vi "IBM4_Diff_Read(I1).vi"(8 "error in":errorcluster, 9 "Neg-Chan":i32=1, 10 "Pos-Chan":i32, 11 "COM resource in":refnum<visa-resource-name>="COM9") -> (0 "error out":errorcluster, 2 "output":i32, 3 "COM resource out":refnum<visa-resource-name>)   [LabVIEW 2021, in "IBM4.lvlib"]
doc: "This VI interfaces with the IBM4 to perform a differential read operation.\n\nThe input channels must be between 0 and 4, while the output will in binary format (thus, integer).\nOnly a single read operation is made with this VI. \n\nAlternate read operations exist covering binary or floating point, single reading, multiple readings, and an average of multiple readings (floating point only)."
uses:
  IBM4.lvlib
  <vilib>/Instr/_visa.llb/VISA Configure Serial Port (Instr).vi
panel:
  out "error out 2":errorcluster
  out "read buffer":string
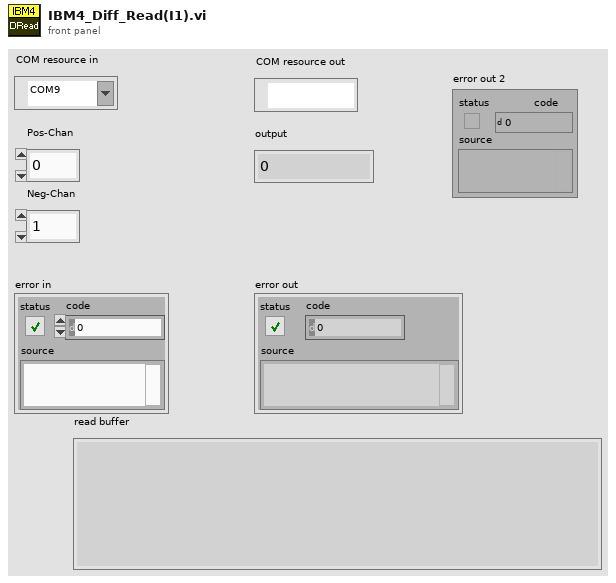
[diagram p1: front panel]
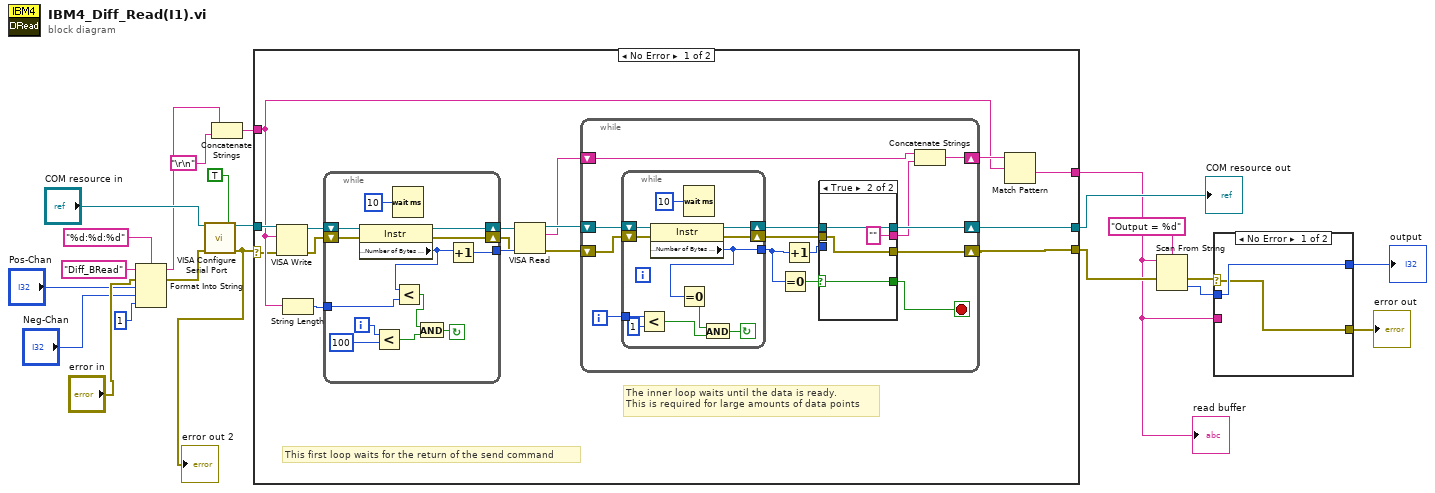
[diagram p0: block diagram]
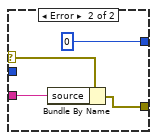
[diagram p2: hidden frame]
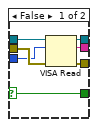
[diagram p3: hidden frame]
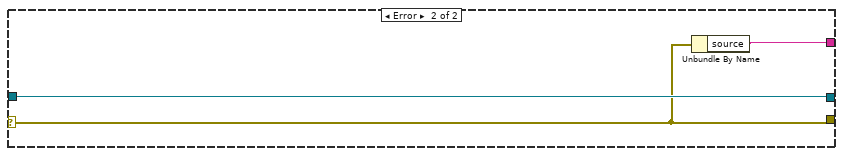
[diagram p4: hidden frame]
diagram:
  n1 = Format Into String(format string="%d:%d:%d", initial string="Diff_BRead", error in="error in", "Pos-Chan", "Neg-Chan", 1 ("input 2")) -> (resulting string=w9:string, error out=w18:errorcluster)
  n2 = call-poly "VISA Configure Serial Port"("VISA resource name"="COM resource in", "Enable Termination\nChar (T)"=TRUE ("Enable Termination\nChar (T)"), "error in (no error)"=w18) -> ("VISA resource name out"=w15:refnum<visa-resource-name>, "error out"=w14:errorcluster)  [unwired: 11 in]
  "error out 2" <- w14
  n3 = Concatenate Strings(w9, "\r\n") -> (w8:string)
  n4 = case shown="No Error" w14 {
    selector: w14 -> [w25 w88]
    tunnel: w15 -> [w38 w90]
    tunnel: [w24 w88] -> w12
    tunnel: [w36 w89] -> w4
    tunnel: w8 -> [w35 _]
    tunnel: [w23 w90] -> w13
    frame No Error {
      # "The inner loop waits until the data is ready.\nThis is required for large amounts of data points"
      # "This first loop waits for the return of the send command"
      n5 = VISA Write(VISA resource name=w38, write buffer=w35, error in (no error)=w25) -> (VISA resource name out=w34:refnum<visa-resource-name>, error out=w33:errorcluster)  [unwired: 1 out]
      n6 = String Length(string=w35) -> (length=w26:i32)
      n7 = while {
        tunnel: [w40] -> w31
        shift-right: [w50] -> w32
        shift-left: w34 -> [w51]
        shift-right: [w48] -> w30
        shift-left: w33 -> [w49]
        tunnel: w26 -> [w46]
        i -> [w41]
        stop <- w44 continue-if-true
        n8 = property class="Instr"(reference=w51, error in=w49) -> (reference out=w50:refnum<visa-resource-name>, error out=w48:errorcluster, "Serial Settings:Number of Bytes at Serial Port"=w39:u32)
        n9 = Less?(x=w41, y=100) -> (x < y?=w43:bool)
        n10 = Wait (ms)(milliseconds to wait=u32 10) -> ()  [unwired: 1 out]
        n11 = Less?(x=w39, y=w46) -> (x < y?=w42:bool)
        n12 = And(x=w42, y=w43) -> (x .and. y?=w44:bool)
        n13 = Increment(x=w39) -> (x+1=w40:u32)
      }
      n14 = VISA Read(VISA resource name=w32, byte count=w31, error in (no error)=w30) -> (VISA resource name out=w29:refnum<visa-resource-name>, read buffer=w27:string, error out=w28:errorcluster)  [unwired: 1 out]
      n15 = while {
        shift-right: [w65] -> w23
        shift-left: w29 -> [w63]
        shift-right: [w64] -> w24
        shift-left: w28 -> [w61]
        shift-right: [w59] -> w37
        shift-left: w27 -> [w57]
        i -> [w56]
        stop <- w52 stop-if-true
        n16 = while {
          tunnel: [w82] -> w55
          shift-right: [w86] -> w62
          shift-left: w63 -> [w87]
          shift-right: [w84] -> w60
          shift-left: w61 -> [w85]
          tunnel: w56 -> [w81]
          stop <- w79 continue-if-true
          n17 = Less?(x=w81, y=1) -> (x < y?=w78:bool)
          n18 = property class="Instr"(reference=w87, error in=w85) -> (reference out=w86:refnum<visa-resource-name>, error out=w84:errorcluster, "Serial Settings:Number of Bytes at Serial Port"=w82:u32)
          n19 = Equal To 0?(x=w82) -> (x = 0?=w77:bool)
          n20 = Wait (ms)(milliseconds to wait=u32 10) -> ()  [unwired: 1 out]
          n21 = And(x=w77, y=w78) -> (x .and. y?=w79:bool)
        }
        n22 = Equal To 0?(x=w55) -> (x = 0?=w53:bool)
        n23 = Increment(x=w55) -> (x+1=w54:u32)
        n24 = case shown="True" w53 {
          selector: w53 -> [w66 w75]
          tunnel: [w72 w76] -> w65
          tunnel: [w71 w74] -> w64
          tunnel: w62 -> [w70 w76]
          tunnel: w60 -> [w69 w74]
          tunnel: [w68 "" ("read buffer")] -> w58
          tunnel: w54 -> [w67 _]
          tunnel: [w66 w75] -> w52
          frame False {
            n25 = VISA Read(VISA resource name=w70, byte count=w67, error in (no error)=w69) -> (VISA resource name out=w72:refnum<visa-resource-name>, read buffer=w68:string, error out=w71:errorcluster)  [unwired: 1 out]
          }
          frame True {
          }
        }
        n26 = Concatenate Strings(w57, w58) -> (w59:string)
      }
      n27 = Match Pattern(string=w37, regular expression=w35) -> (after substring=w36:string)  [unwired: 1 in, 3 out]
    }
    frame Error {
      n28 = Unbundle By Name(w88) -> ("source"=w89:string)
    }
  }
  "COM resource out" <- w13
  "read buffer" <- w4
  n29 = Scan From String(format string="Output = %d", input string=w4, error in=w12) -> (error out=w7:errorcluster, output 1=w1:i32)  [unwired: 2 in, 2 out]
  n30 = case shown="No Error" w7 {
    selector: w7 -> [w91 w95]
    tunnel: w1 -> [w92 _]
    tunnel: [w92 0] -> w6
    tunnel: [w91 w93] -> w5
    tunnel: w4 -> [_ w94]
    frame No Error {
    }
    frame Error {
      n31 = Bundle By Name(cluster=w95, "source"=w94) -> (w93:errorcluster)
    }
  }
  "error out" <- w5
  "output" <- w6
